vi "Read Ref.vi"(4 "User Parameter":cluster{refnum<vi>, refnum<vi>}, 6 "Point List":refnum<vi>, 7 "Event Common Data":cluster{"Source":T1, "Type":T2, "Time":u32} {"Source" items=["LabVIEW UI"=0, "ActiveX"=1, "User Event"=25]}) -> ()   [LabVIEW 2015]
uses:
  <vilib>/event_ctls.llb/eventsource.ctl
  <vilib>/event_ctls.llb/lveventtype.ctl
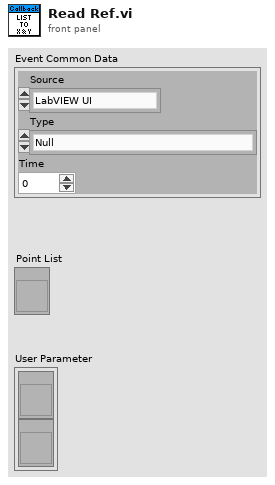
[diagram p1: front panel]
types:
  T1 = typedef "eventsource.ctl" = u32
  T2 = typedef "lveventtype.ctl" = enum32{"Null", "Timeout", "Annotation Menu Selection", "Annotation Menu Selection?", "App Instance Close", "App Instance Close?", "Autoscale Range Change", "Bookmark Info Change", "Cell Edit", "Cell Edit?", "Cursor Grab", "Cursor Grab?", "Cursor Menu Selection", "Cursor Menu Selection?", "Cursor Move", "Cursor Release", "Data Change", "Direction Change", "Display State Change", "Drag Ended", "Drag Enter", "Drag Leave", "Drag Over", "Drag Source Update", "Drag Starting", "Drag Starting?", "Drop", "Exec State Change", "Key Down", "Key Down?", "Key Repeat", "Key Repeat?", "Key Up", "Listbox Double Click", "Menu Activation?", "Menu Selection (App)", "Menu Selection? (App)", "Menu Selection (User)", "Mouse Down", "Mouse Down?", "Mouse Enter", "Mouse Leave", "Mouse Move", "Mouse Up", "Mouse Wheel", "NI Security User Change (App)", "Pane Size", "Panel Close", "Panel Close?", "Panel Resize", "Plot Attribute Change", "Scale Range Change", "Shortcut Menu Activation?", "Shortcut Menu Selection (App)", "Shortcut Menu Selection? (App)", "Shortcut Menu Selection (User)", "Tree Double Click", "Tree Drag", "Tree Drag?", "Tree Drop", "Tree Drop?", "Tree Item Close", "Tree Item Close?", "Tree Item Open", "Tree Item Open?", "User Event", "Value Change"}
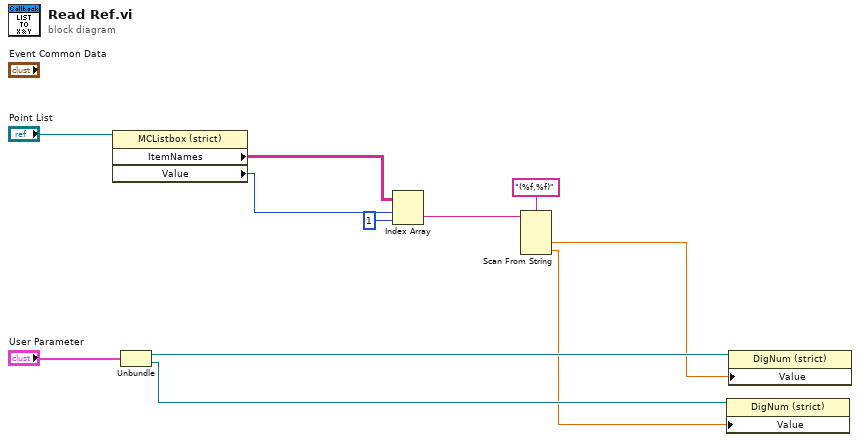
[diagram p0: block diagram]
diagram:
  n1 = property class="MCListbox (strict)"(reference="Point List") -> ("ItemNames"=w10:string[][], "Value"=w9:i32)  [unwired: 1 in, 2 out]
  n2 = Unbundle("User Parameter") -> (w6:refnum<vi>, w5:refnum<vi>)
  n3 = Index Array(array=w10, index (row)=w9, index (col)=1 ("disabled index (col)")) -> (element=w4:string)
  n4 = Scan From String(format string="(%f,%f)", input string=w4) -> (output 1=w1:dbl, output 2=w2:dbl)  [unwired: 4 in, 3 out]
  n5 = property class="DigNum (strict)"(reference=w5, "Value"=w2) -> ()  [unwired: 1 in, 2 out]
  n6 = property class="DigNum (strict)"(reference=w6, "Value"=w1) -> ()  [unwired: 1 in, 2 out]
